vi "Raster Array.vi"(0 "Initial Vx":dbl, 1 "Final Vx":dbl, 2 "x rows":dbl, 3 "Initial Vy":dbl, 4 "Final Vy":dbl, 5 "y columns":dbl) -> (14 "X Array":dbl[](array[numeric]), 19 "Y Array":dbl[](array[numeric]))   [LabVIEW 2014]
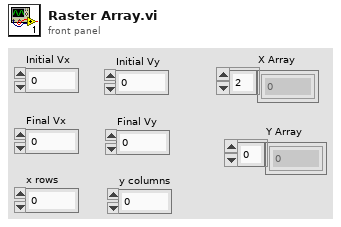
[diagram p1: front panel]
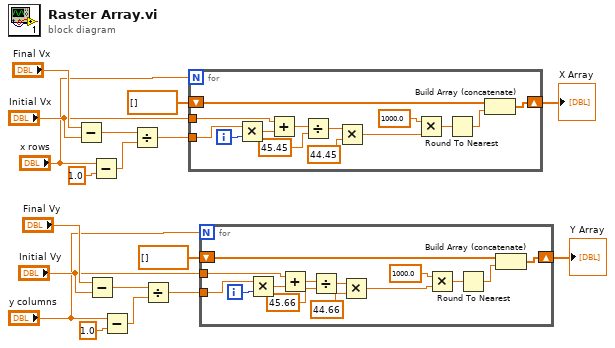
[diagram p0: block diagram]
diagram:
  n1 = Subtract(x="Final Vx", y="Initial Vx") -> (x-y=w16:dbl)
  n2 = Subtract(x="Final Vy", y="Initial Vy") -> (x-y=w7:dbl)
  n3 = Subtract(x="x rows", y=1.0) -> (x-y=w15:dbl)
  n4 = Subtract(x="y columns", y=1.0) -> (x-y=w12:dbl)
  n5 = Divide(x=w16, y=w15) -> (x/y=w14:dbl)
  n6 = Divide(x=w7, y=w12) -> (x/y=w11:dbl)
  n7 = for {
    N: "x rows" -> [_]
    tunnel: w14 -> [w32]
    tunnel: "Initial Vx" -> [w29]
    shift-right: [w26] -> w2
    shift-left: dbl[] [] -> [w28]
    i -> [w31]
    n8 = Multiply(x=w32, y=w31) -> (x*y=w30:dbl)
    n9 = Add(x=w29, y=w30) -> (x+y=w23:dbl)
    n10 = Divide(x=w23, y=45.45) -> (x/y=w22:dbl)
    n11 = Multiply(x=w22, y=44.45) -> (x*y=w21:dbl)
    n12 = Multiply(x=1000.0, y=w21) -> (x*y=w25:dbl)
    n13 = Round To Nearest(number=w25) -> (nearest integer value=w24:dbl)
    n14 = Build Array (concatenate)(w28, w24) -> (w26:dbl[])
  }
  "X Array" <- w2
  n15 = for {
    N: "y columns" -> [_]
    tunnel: w11 -> [w45]
    tunnel: "Initial Vy" -> [w43]
    shift-right: [w40] -> w1
    shift-left: dbl[] [] -> [w42]
    i -> [w46]
    n16 = Multiply(x=w45, y=w46) -> (x*y=w44:dbl)
    n17 = Add(x=w43, y=w44) -> (x+y=w37:dbl)
    n18 = Divide(x=w37, y=45.66) -> (x/y=w36:dbl)
    n19 = Multiply(x=w36, y=44.66) -> (x*y=w35:dbl)
    n20 = Multiply(x=1000.0, y=w35) -> (x*y=w39:dbl)
    n21 = Round To Nearest(number=w39) -> (nearest integer value=w38:dbl)
    n22 = Build Array (concatenate)(w42, w38) -> (w40:dbl[])
  }
  "Y Array" <- w1
